vi "Calc min points to read.vi"(3 "error in":errorcluster, 4 "Target number of points":u64, 5 "Logging queue element":T1={"Imaging Protocol"=enum."Live Imaging", "Number of Trials"=0, "Frame Size"=512, "# Averaged frames"=0, "Dwell time (us)"=0.0, "Index of Z-plane"=0, "Timelapse?"=FALSE, "Logging process is active"=FALSE, "Speed logging enabled"=FALSE, "tdms file ref"=refnum, "path"=path "", "Trial Number"=0, "Expected # points acquired"=FALSE, "Manually stopped"=FALSE, "Ch0 data"=[], "Ch1 data"=[], "Ref Data"=[], "Last trial"=FALSE, "Ref Dwell time (us)"=0.0, "# Ref Averaged frames"=0, "Ref X Length"=0, "Ref Y Length"=0, "Points acquired"={"Ch0 last trial"=0, "Ch1 last trial"=0, "All trials"=0}} {"Ref Dwell time (us)" format="%#.6g"; "Frame Size" items=["100X100"=100, "128X128"=128, "200X200"=200, "256X256"=256, "512X512"=512, "1024x1024"=1024, "2048x2048"=2048]; "Dwell time (us)" format="%#.6g"}) -> (0 "error out":errorcluster, 1 "Read at least # Ref points":u32, 2 "Read at least # points":u32)   [LabVIEW 2017]
uses:
  Typedefs/Logging queue element.ctl
  Typedefs/Imaging Protocols enum.ctl
  Typedefs/Frame Size.ctl
  Typedefs/Acquired points count.ctl
  Global Variables/General Globals.vi
panel:
  in  "Very important value":u64=200000
  in  "Ref Point multiplier":u16=1
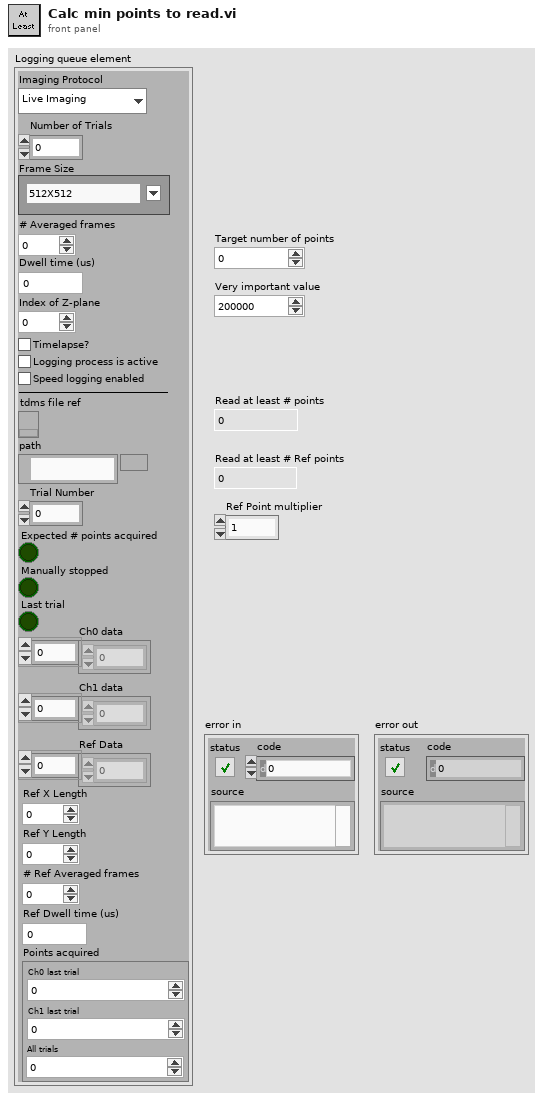
[diagram p1: front panel]
types:
  T1 = typedef "Logging queue element.ctl" = cluster{"Imaging Protocol":T2, "Number of Trials":u16, "Frame Size":T3, "# Averaged frames":u16, "Dwell time (us)":dbl, "Index of Z-plane":i32, "Timelapse?":bool, "Logging process is active":bool, "Speed logging enabled":bool, "tdms file ref":refnum<k34>, "path":path, "Trial Number":i32, "Expected # points acquired":bool, "Manually stopped":bool, "Ch0 data":u32[], "Ch1 data":u32[], "Ref Data":u32[], "Last trial":bool, "Ref Dwell time (us)":dbl, "# Ref Averaged frames":u16, "Ref X Length":u16, "Ref Y Length":u16, "Points acquired":T4}
  T2 = typedef "Imaging Protocols enum.ctl" = enum16{"AOL Z-Stack", "Motor Z Stack", "Functional Acquisition", "Single Plane Acquisition", "Volume Acquisition", "Live Imaging", "Live Plane Imaging", "Live Volume Imaging"}
  T3 = typedef "Frame Size.ctl" = u16
  T4 = typedef "Acquired points count.ctl" = cluster{"Ch0 last trial":u64, "Ch1 last trial":u64, "All trials":u64}
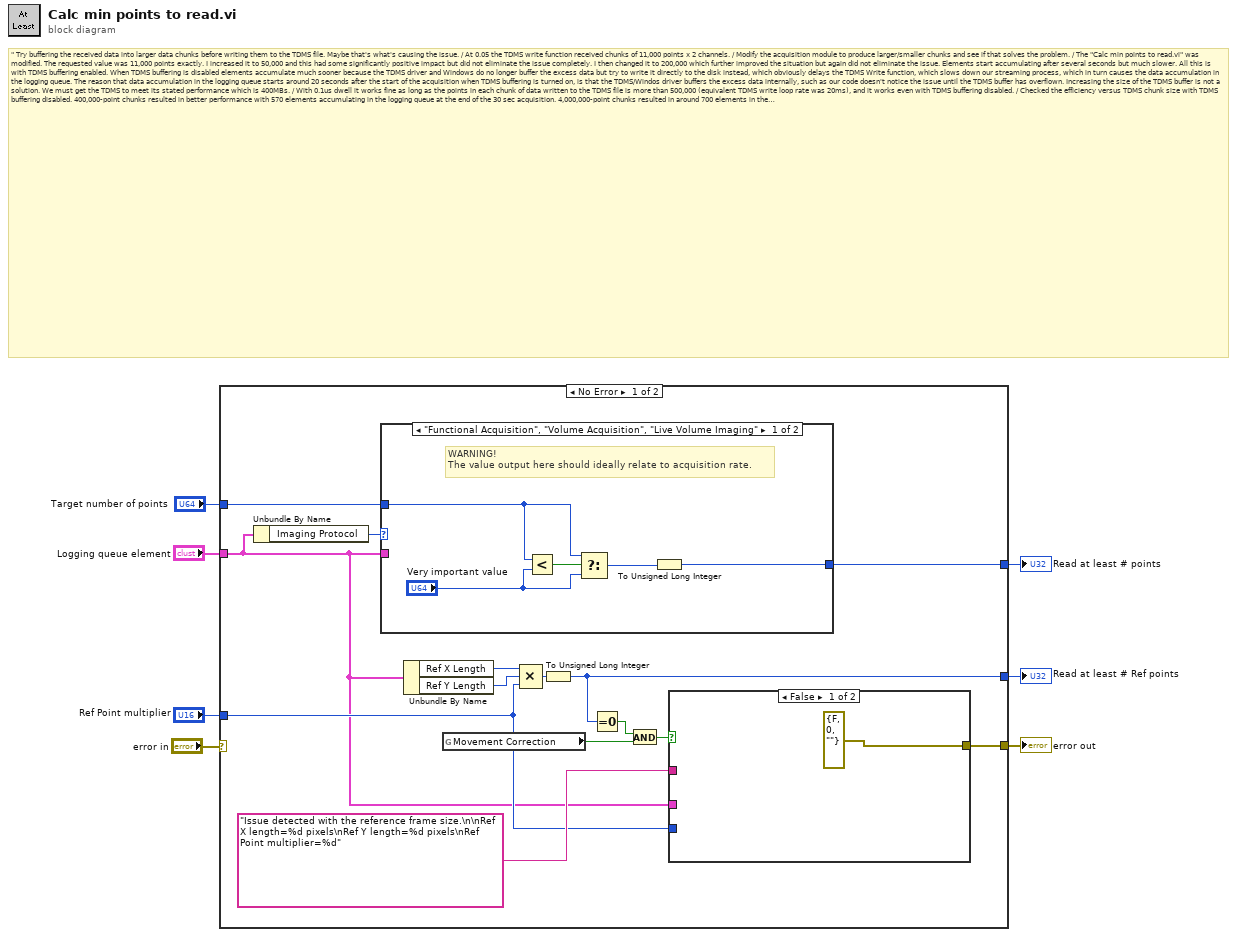
[diagram p0: block diagram]
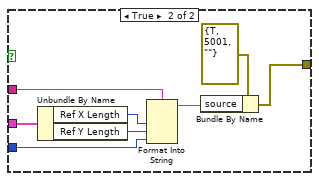
[diagram p2: hidden frame]
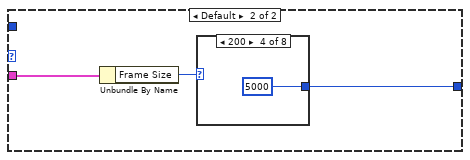
[diagram p3: hidden frame]
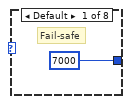
[diagram p4: hidden frame]
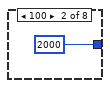
[diagram p5: hidden frame]
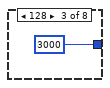
[diagram p6: hidden frame]
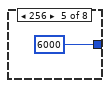
[diagram p7: hidden frame]
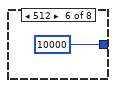
[diagram p8: hidden frame]
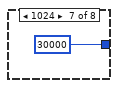
[diagram p9: hidden frame]
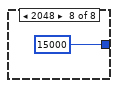
[diagram p10: hidden frame]
diagram:
  # "\"\tTry buffering the received data into larger data chunks before writing them to the TDMS file. Maybe that's what's causing the issue. / At 0.05 the TDMS write function received chunks of 11,000 points x 2 channels. / Modify the acquisition module to produce larger/smaller chunks and see if that solves the problem. / The \"Calc min points to read.vi\" was modified. The requested value was 11,000 points exactly. I increased it to 50,000 and this had some significantly positive impact but did not eliminate the issue completely. I then changed it to 200,000 which further improved the situation but again did not eliminate the issue. Elements start accumulating after several seconds but much slower. All this is with TDMS buffering enabled. When TDMS buffering is disabled elements accumulate much sooner because the TDMS driver and Windows do no longer buffer the excess data but try to write it directly to the disk instead, which obviously delays the TDMS Write function, which slows down our streaming process, which in turn causes the data accumulation in the logging queue. The reason that data accumulation in the logging queue starts around 20 seconds after the start of the acquisition when TDMS buffering is turned on, is that the TDMS/Windos driver buffers the excess data internally, such as our code doesn't notice the issue until the TDMS buffer has overflown. Increasing the size of the TDMS buffer is not a solution. We must get the TDMS to meet its stated performance which is 400MBs. / With 0.1us dwell it works fine as long as the points in each chunk of data written to the TDMS file is more than 500,000 (equivalent TDMS write loop rate was 20ms), and it works even with TDMS buffering disabled. / Checked the efficiency versus TDMS chunk size with TDMS buffering disabled. 400,000-point chunks resulted in better performance with 570 elements accumulating in the logging queue at the end of the 30 sec acquisition. 4,000,000-point chunks resulted in around 700 elements in the queue (note each element contained 4 Million points) as compared to the previous case where each element contained just 400,000 points). With 4,000-point chunks there were over 10,000 points in the queue before an error occurred. With 40,000-point chunks the queue size reached 3500 elements.\n4,000,000 -> 700 ' 2800M points in the queue\n400,000   -> 570 ' 228M points in the queue\n300,000  -> 600 ' 180M points\n200,000   -> 550  ' 110M points\n100,000   -> 2100 ' 210M points\n40,000    -> 3500 ' 140M points\n4,000      -> >10,000 ' N/A\nI set the chunk size to 200,000 points at least for now since it appears to be the most optimal value."
  n1 = case shown="No Error" "error in" {
    selector: "error in" -> [_ w47]
    tunnel: [w21 _] -> w7
    tunnel: "Ref Point multiplier" -> [w9 _]
    tunnel: "Logging queue element" -> [w8 _]
    tunnel: "Target number of points" -> [w16 _]
    tunnel: [w13 _] -> w3
    tunnel: [w11 w47] -> w2
    frame No Error {
      n2 = Unbundle By Name(w8) -> ("Imaging Protocol"=w17:T2)
      n3 = case shown="\"Functional Acquisition\", \"Volume Acquisition\", \"Live Volume Imaging\"" w17 {
        tunnel: [w31 w38] -> w21
        tunnel: w8 -> [_ w36]
        tunnel: w16 -> [w34 _]
        frame "Functional Acquisition", "Volume Acquisition", "Live Volume Imaging" {
          # "WARNING!\nThe value output here should ideally relate to acquisition rate."
          n4 = Less?(x=w34, y="Very important value") -> (x < y?=w35:bool)
          n5 = Select(t=w34, s=w35, f="Very important value") -> (s? t:f=w32:u64)
          n6 = To Unsigned Long Integer(number=w32) -> (unsigned 32bit integer=w31:u32)
        }
        frame Default {
          n7 = Unbundle By Name(w36) -> ("Frame Size"=w37:T3)
          n8 = case shown="200" w37 {
            tunnel: [u32 7000 ("unsigned 32bit integer") u32 2000 ("unsigned 32bit integer") u32 3000 ("unsigned 32bit integer") u32 5000 ("unsigned 32bit integer") u32 6000 ("unsigned 32bit integer") u32 10000 ("unsigned 32bit integer") u32 30000 ("unsigned 32bit integer") u32 15000 ("unsigned 32bit integer")] -> w38
            frame Default {
              # "Fail-safe"
            }
            frame 100 {
            }
            frame 128 {
            }
            frame 200 {
            }
            frame 256 {
            }
            frame 512 {
            }
            frame 1024 {
            }
            frame 2048 {
            }
          }
        }
      }
      n9 = Unbundle By Name(w8) -> ("Ref X Length"=w20:u16, "Ref Y Length"=w19:u16)
      n10 = global read "General Globals.vi" "Movement Correction"() -> (w15:bool)
      n11 = Compound Arithmetic op=MULTIPLY(w20, w19, w9) -> (w18:u16)
      n12 = To Unsigned Long Integer(number=w18) -> (unsigned 32bit integer=w13:u32)
      n13 = Equal To 0?(x=w13) -> (x = 0?=w14:bool)
      n14 = And(x=w14, y=w15) -> (x .and. y?=w12:bool)
      n15 = case shown="False" w12 {
        tunnel: [errorcluster {"status"=FALSE, "code"=0, "source"=""} ("error out") w29] -> w11
        tunnel: "Issue detected with the reference frame size.\n\nRef X length=%d pixels\nRef Y length=%d pixels\nRef Point multiplier=%d" ("source") -> [_ w27]
        tunnel: w9 -> [_ w26]
        tunnel: w8 -> [_ w25]
        frame False {
        }
        frame True {
          n16 = Unbundle By Name(w25) -> ("Ref X Length"=w24:u16, "Ref Y Length"=w23:u16)
          n17 = Format Into String(format string=w27, w24, w23, w26) -> (resulting string=w28:string)  [unwired: 2 in, 1 out]
          n18 = Bundle By Name(cluster=errorcluster {"status"=TRUE, "code"=5001, "source"=""} ("error out"), "source"=w28) -> (w29:errorcluster)
        }
      }
    }
    frame Error {
    }
  }
  "Read at least # points" <- w7
  "Read at least # Ref points" <- w3
  "error out" <- w2
